vi "HFRR ADV v014 new software.vi"() -> ()   [LabVIEW 2025] (continued)
            n3067 = Concatenate Strings("7)" ("string"), w3910) -> (w3911:string)
            n3068 = Concatenate Strings("8)" ("string"), w3907) -> (w3908:string)
            n3069 = local read "HCF 2"() -> (w3946:dbl)
            n3070 = local read "AVP 2"() -> (w3963:dbl)
            n3071 = local read "s.NO"() -> (w3905:string)
            n3072 = call <vilib>:"New Report.vi"("report type"=enum16{"Standard Report", "HTML"}."Standard Report") -> ("report out"=w3984:refnum<class "NI_report.lvclass">, "error out"=w3983:errorcluster)  [unwired: 13 in]
            n3073 = local read "TITTLE"() -> (w3936:string)
            n3074 = Concatenate Strings(w3961, w3904, w3905, w3961, w3939, w3934, w3961, w3938, w3935, w3961, w3940, w3937, w3961) -> (w3954:string)
            "test by" <- w3954
            n3075 = Number To Fractional String(number=w3960, width (-)=i16 6, precision (6)=i16 2) -> (F-format string=w3949:string)  [unwired: 1 in]
            n3076 = Number To Fractional String(number=w3959, width (-)=i16 6, precision (6)=i16 2) -> (F-format string=w3962:string)  [unwired: 1 in]
            n3077 = Number To Fractional String(number=w3975, width (-)=i16 6, precision (6)=i16 2) -> (F-format string=w3980:string)  [unwired: 1 in]
            n3078 = Number To Fractional String(number=w3964, width (-)=i16 6, precision (6)=i16 2) -> (F-format string=w3966:string)  [unwired: 1 in]
            n3079 = Number To Fractional String(number=w3950, width (-)=i16 6, precision (6)=i16 2) -> (F-format string=w3951:string)  [unwired: 1 in]
            n3080 = Number To Fractional String(number=w3963, width (-)=i16 6, precision (6)=i16 2) -> (F-format string=w3965:string)  [unwired: 1 in]
            n3081 = Number To Fractional String(number=w3946, width (-)=i16 6, precision (6)=i16 2) -> (F-format string=w3945:string)  [unwired: 1 in]
            n3082 = Number To Fractional String(number=w3942, precision (6)=i16 2) -> (F-format string=w3941:string)  [unwired: 2 in]
            n3083 = call-dynamic "Set Report Header Text.vi"("report in"=w3984, "center header text"=w3936, "error in (no error)"=w3983) -> ("report out"=w3955:refnum<class "NI_report.lvclass">, "error out"=w3956:errorcluster)  [unwired: 11 in]
            n3084 = Concatenate Strings(w3944, w3928, w3980, w3944, w3925, w3949, w3944, w3923, w3962, w3944, w3920, w3951, w3944, w3916, w3966, w3944, w3913, w3965, w3944, w3911, w3945, w3944, w3908, w3941) -> (w3932:string)
            "export 2" <- w3932
            n3085 = call-poly <vilib>:"Append Report Text.vi"("report in"=w3955, "text"=w3954, "error in (no error)"=w3956) -> ("report out"=w3958:refnum<class "NI_report.lvclass">, "error out"=w3957:errorcluster)  [unwired: 9 in, 2 out]
            n3086 = local read "test by"() -> (w3931:string)
            n3087 = local read "TITTLE"() -> (w3933:string)
            n3088 = call-poly <vilib>:"Append Report Text.vi"("report in"=w3958, "error in (no error)"=w3957) -> ("report out"=w3979:refnum<class "NI_report.lvclass">, "error out"=w3977:errorcluster)  [unwired: 10 in, 2 out]
            n3089 = Concatenate Strings(w3933, w3932, w3931) -> (→"output":string)
            n3090 = call-poly <vilib>:"Append Report Text.vi"("report in"=w3979, "text"=w3932, "error in (no error)"=w3977) -> ("report out"=w3978:refnum<class "NI_report.lvclass">, "error out"=w3976:errorcluster)  [unwired: 9 in, 2 out]
            n3091 = call-dynamic "Print Report.vi"("report in"=w3978, "printer name (default)"=w3986, "error in (no error)"=w3976) -> ("report out"=w3988:refnum<class "NI_report.lvclass">, "error out"=w3989:errorcluster)  [unwired: 11 in]
            n3092 = call-dynamic "Dispose Report.vi"("report in"=w3988, "error in (no error)"=w3989) -> ()  [unwired: 13 in, 1 out]
          }
        }
        n3093 = case shown="True" "Print 2" {
          frame False {
          }
          frame True {
            n3094 = flat-sequence {
              frame #0 {
                n3095 = local read "s.NO"() -> (→"s.NO 2":string)
                n3096 = Wait (ms)(milliseconds to wait=u32 20) -> ()  [unwired: 1 out]
                n3097 = local read "Sample ID  3"() -> (→"Sample ID  6":string)
                n3098 = local read "Sample ID  4"() -> (→"Sample ID  7":string)
                n3099 = local read "Sample ID"() -> (→"Sample ID  2":string)
                n3100 = local read "Tested by"() -> (→"Tested by 2":string)
                n3101 = local read "Test Date"() -> (→"Test Date 2":string)
                n3102 = local read "Humidity after test 3"() -> (→"Humidity after test 4":dbl)
                n3103 = local read "Ref A Test Date :"() -> (→"TITTLE 4":string)
                n3104 = local read "Temperature before test 3"() -> (w3811:dbl)
                n3105 = local read "Temperature before test 3"() -> (→"Temperature after test 5":dbl)
                n3106 = local read "Temperature after test 3"() -> (→"Temperature after test 4":dbl)
                n3107 = local read "Humidity before test 3"() -> (→"Humidity before test 4":dbl)
                n3108 = local write "Temperature before test 3"(w3811) -> ()
                n3109 = local read "image data"() -> (w3802:T16)
                n3110 = String To Path(string="C:\\LAB-IQ\\im\\Temp_resized.jpg") -> (path=w3803:path)
                "path 2" <- w3803
                n3111 = call <vilib>:"Write JPEG File.vi"("image data"=w3802, "path to JPEG file"=w3803) -> ()  [unwired: 8 in, 2 out]
                "Ref A Test Date :" <- "Ref A Test Date :"
                "Ref B Test Date :" <- "Ref B Test Date :"
                "Ref B Scar Value :" <- "Ref B Scar Value :"
                "Ref A Scar Value :" <- "Ref A Scar Value :"
              }
              frame #1 {
                (unwired) HTML_Report_Image_Alignment."MIDDLE" ("alignment (default)")
                w3839 = u16 0 items=["portrait", "landscape"] ("orientation (portrait)")
                (unwired) HTML_Report_Image_Alignment."ABSMIDDLE" ("alignment (default)")
                (unwired) "TESTED BY : "
                (unwired) "TESTED DATE :"
                (unwired) "SAMPLE ID : "
                (unwired) "SAMPLE DESIGN : "
                w3872 = "\r"
                # "add image"
                n3112 = Wait (ms)(milliseconds to wait=u32 20) -> ()  [unwired: 1 out]
                n3113 = local read "Sample ID  2"() -> (w3865:string)
                n3114 = local read "Wear Scar X"() -> (w3837:dbl)
                "Length ( microns ) 2" <- w3837
                n3115 = local read "Wear Scar Y"() -> (w3836:dbl)
                "Wear Scar Y ( microns ) :" <- w3836
                n3116 = local read "Test Date 2"() -> (w3866:string)
                n3117 = local read "Tested by 2"() -> (w3867:string)
                n3118 = local read "String 46"() -> (w3863:string)
                n3119 = local read "String 48"() -> (w3869:string)
                n3120 = local read "String 47"() -> (w3868:string)
                n3121 = local read "String 49"() -> (w3870:string)
                n3122 = local read "String 10"() -> (w3823:string)
                n3123 = local read "s.NO 2"() -> (w3864:string)
                n3124 = Add(x=w3837, y=w3836) -> (x+y=w3835:dbl)
                n3125 = call <vilib>:"New Report.vi"("report type"=enum16{"Standard Report", "HTML"}."HTML") -> ("report out"=w3843:refnum<class "NI_report.lvclass">, "error out"=w3841:errorcluster)  [unwired: 13 in]
                n3126 = Concatenate Strings(w3872, w3863, w3864, w3872, w3869, w3865, w3872, w3868, w3866, w3872, w3870, w3867, w3872) -> (→"test by 2":string)
                n3127 = Concatenate Strings("C:\\LAB-IQ\\Data\\" ("string"), w3823, ".jpg" ("string")) -> ()  [unwired: 1 out]
                n3128 = Divide(x=w3835, y=2.0) -> (x/y=→"Mean Wear ( microns) :":dbl)
                n3129 = call-dynamic "Set Report Orientation.vi"("report in"=w3843, "orientation (portrait)"=w3839, "error in (no error)"=w3841) -> ("report out"=w3842:refnum<class "NI_report.lvclass">, "error out"=w3840:errorcluster)  [unwired: 11 in]
                n3130 = for {
                  N: 5 -> [_]
                  tunnel: w3842 -> [w3893]
                  tunnel: [w3892] -> w3821
                  tunnel: w3840 -> [w3891]
                  tunnel: [w3890] -> w3820
                  n3131 = call-dynamic "Set Report Tab Width.vi"("report in"=w3893, "error in (no error)"=w3891) -> ("report out"=w3892:refnum<class "NI_report.lvclass">, "error out"=w3890:errorcluster)  [unwired: 12 in]
                }
                n3132 = local read "TITTLE"() -> (w3838:string)
                n3133 = call-dynamic "Set Report Header Text.vi"("report in"=w3821, "center header text"=w3838, "error in (no error)"=w3820) -> ("report out"=w3859:refnum<class "NI_report.lvclass">, "error out"=w3858:errorcluster)  [unwired: 11 in]
                n3134 = for {
                  N: 1 -> [_]
                  tunnel: [w3897] -> w3845
                  tunnel: [w3896] -> w3844
                  tunnel: w3859 -> [w3895]
                  tunnel: w3858 -> [w3894]
                  n3135 = call-dynamic "New Report Line.vi"("report in"=w3895, "error in (no error)"=w3894) -> ("report out"=w3897:refnum<class "NI_report.lvclass">, "error out"=w3896:errorcluster)  [unwired: 12 in]
                }
                n3136 = for {
                  N: 2 -> [_]
                  tunnel: [w3889] -> w3851
                  tunnel: [w3888] -> w3850
                  tunnel: w3845 -> [w3887]
                  tunnel: w3844 -> [w3886]
                  n3137 = call-dynamic "New Report Line.vi"("report in"=w3887, "error in (no error)"=w3886) -> ("report out"=w3889:refnum<class "NI_report.lvclass">, "error out"=w3888:errorcluster)  [unwired: 12 in]
                }
                n3138 = for {
                  N: 25 -> [_]
                  tunnel: w3851 -> [w3885]
                  tunnel: w3850 -> [w3883]
                  tunnel: [w3884] -> w3854
                  tunnel: [w3882] -> w3853
                  n3139 = call-dynamic "Set Report Tab Width.vi"("report in"=w3885, "error in (no error)"=w3883) -> ("report out"=w3884:refnum<class "NI_report.lvclass">, "error out"=w3882:errorcluster)  [unwired: 12 in]
                }
                n3140 = control-ref of="Tab Control 9"() -> (w3849:refnum<vi>)
                n3141 = call-dynamic "Append Control Image to Report.vi"("report in"=w3854, "alignment (default)"=HTML_Report_Image_Alignment."ABSMIDDLE", "ctrl reference"=w3849, "error in (no error)"=w3853) -> ("report out"=w3848:refnum<class "NI_report.lvclass">, "error out"=w3847:errorcluster)  [unwired: 8 in, 2 out]
                n3142 = for {
                  N: 3 -> [_]
                  tunnel: [w3881] -> w3832
                  tunnel: [w3880] -> w3831
                  tunnel: w3848 -> [w3879]
                  tunnel: w3847 -> [w3878]
                  n3143 = call-dynamic "New Report Line.vi"("report in"=w3879, "error in (no error)"=w3878) -> ("report out"=w3881:refnum<class "NI_report.lvclass">, "error out"=w3880:errorcluster)  [unwired: 12 in]
                }
                n3144 = for {
                  N: 100 -> [_]
                  tunnel: w3832 -> [w3877]
                  tunnel: w3831 -> [w3875]
                  tunnel: [w3876] -> w3828
                  tunnel: [w3874] -> w3826
                  n3145 = call-dynamic "Set Report Tab Width.vi"("report in"=w3877, "error in (no error)"=w3875) -> ("report out"=w3876:refnum<class "NI_report.lvclass">, "error out"=w3874:errorcluster)  [unwired: 12 in]
                }
                n3146 = String To Path(string="C:\\LAB-IQ\\im\\Temp_resized.jpg") -> (path=w3818:path)
                n3147 = call-poly <vilib>:"Append Image to Report.vi"("report in"=w3828, "path or URL of image"=w3818, "error in (no error)"=w3826) -> ("report out"=w3827:refnum<class "NI_report.lvclass">, "error out"=w3825:errorcluster)  [unwired: 9 in, 2 out]
                n3148 = call-poly <vilib>:"Open HTML Report in Browser.vi"("report in"=w3827, "error in (no error)"=w3825) -> ("report out"=w3862:refnum<class "NI_report.lvclass">, "error out"=w3861:errorcluster)  [unwired: 11 in, 1 out]
                n3149 = call-dynamic "Dispose Report.vi"("report in"=w3862, "error in (no error)"=w3861) -> ()  [unwired: 13 in, 1 out]
              }
              frame #2 {
              }
              frame #3 {
                n3150 = disable-structure shown="Disabled" {
                  frame Disabled {
                    n3151 = local read "String 10"() -> (w3902:string)
                    n3152 = Concatenate Strings("C:\\LAB-IQ-NXT\\Data\\" ("string"), w3902, ".jpg" ("string")) -> (w3900:string)
                    n3153 = String To Path(string=w3900) -> (path=w3899:path)
                    n3154 = Delete(path (use dialog)=w3899) -> ()  [unwired: 4 in, 3 out]
                  }
                  frame Enabled {
                  }
                }
                n3155 = local write "Print 2"(FALSE ("Print")) -> ()
              }
            }
          }
        }
      }
    }
    n3156 = property on="SetTemp" class="DigNum (strict)"("Disabled"=w1838) -> ()  [unwired: 2 in, 2 out]
    n3157 = Multiply(x=w1828, y=w1830) -> (x*y=w1829:dbl)
    n3158 = local read "MWSD"() -> (w1827:dbl)
    n3159 = Add(x=w1829, y=w1827) -> (x+y=→"WS1.4":dbl)
    n3160 = Wait (ms)(milliseconds to wait=u32 50) -> ()  [unwired: 1 out]
    n3161 = Wait (ms)(milliseconds to wait=u32 50) -> ()  [unwired: 1 out]
    n3162 = local read "Quit"() -> (w1826:bool)
  }
  n3163 = VISA Close(VISA resource name=w52, error in (no error)=w51) -> (error out=w49:errorcluster)
  n3164 = call <vilib>:"Clear Errors.vi"("error in (no error)"=w49) -> ()  [unwired: 5 in, 2 out]
  n3165 = VISA Close(VISA resource name=w37, error in (no error)=w36) -> ()  [unwired: 1 out]
  n3166 = while {
    tunnel: [w4063] -> w46
    shift-right: [w4056] -> _
    shift-left: 0.0 -> [w4059]
    shift-right: [w4055] -> _
    shift-left: 0.0 -> [w4058]
    shift-right: [w4054] -> _
    shift-left: 400.0 ("vc_cmd") -> [w4057]
    stop <- w4063 stop-if-true
    # "PID LOGIC"
    n3167 = local read "RUN"() -> (w4061:bool)
    n3168 = local read "Auto Start Temp"() -> (w4050:bool)
    n3169 = local read "Auto Start Test"() -> (w4060:bool)
    n3170 = local read "START TEMP"() -> (w4052:bool)
    n3171 = And(x=w4050, y=w4060) -> (x .and. y?=w4051:bool)
    n3172 = Or(x=w4061, y=w4051) -> (x .or. y?=w4062:bool)
    n3173 = And(x=w4062, y=w4052) -> (x .and. y?=w4053:bool)
    n3174 = Wait (ms)(milliseconds to wait=u32 20) -> ()  [unwired: 1 out]
    n3175 = case shown="True" w4053 {
      tunnel: [400.0 ("out_vc_cmd") w4083] -> w4054
      tunnel: [w4066 w4085] -> w4055
      tunnel: [w4066 w4084] -> w4056
      tunnel: w4059 -> [_ w4074]
      tunnel: w4058 -> [_ w4073]
      tunnel: w4057 -> [_ w4072]
      frame False {
        w4066 = 0.0 ("error_out")
      }
      frame True {
        n3176 = local read "Set Strk"() -> (w4069:dbl)
        n3177 = local read "LVDT STROKE"() -> (w4067:dbl)
        n3178 = Add(x=w4069, y="Add up Stroke") -> (x+y=w4070:dbl)
        n3179 = formula code="// Zero-Hardcode Explicit Positional-Form PID Engine\n// Inputs: target_stroke, measured_stroke, dt, prev_error, integral_accumulator_in, prev_vc_cmd\n//         kp, ki, kd, max_step_change, max_amplitude, min_amplitude, startup_cmd\n// Outputs: vc_cmd, error_out, out_error, integral_accumulator_out, out_vc_cmd\n\n// 1. Calculate Tracking Error\nfloat current_error = target_stroke - measured_stroke;\nerror_out = current_error;\n\n// 2. Compute Proportional Term\nfloat p_term = kp * current_error;\n\n// 3. Compute Derivative Term\nfloat d_term = 0.0;\nif (dt > 0.0) {\n    d_term = kd * ((current_error - prev_error) / dt);\n}\n\n// 4. Update and Accumulate Integral Term\nfloat current_integral = integral_accumulator_in + (current_error * dt);\nfloat i_term = ki * current_integral;\n\n// 5. Calculate Ideal Target Command\nfloat ideal_command = startup_cmd + p_term + i_term + d_term;\n\n// 6. Anti-Windup Protection (Back-calculation method)\nif (ideal_command > max_amplitude) {\n    float excess = ideal_command - max_amplitude;\n    if (ki > 0.0) {\n        current_integral -= excess / ki;\n    }\n    ideal_command = max_amplitude;\n} else if (ideal_command < min_amplitude) {\n    float excess = ideal_command - min_amplitude;\n    if (ki > 0.0) {\n        current_integral -= excess / ki;\n    }\n    ideal_command = min_amplitude;\n}\n\n// 7. Apply Loop Rate Limiting (Protects voice coil from large voltage steps)\nfloat raw_adjustment = ideal_command - prev_vc_cmd;\n\nif (raw_adjustment > max_step_change) {\n    raw_adjustment = max_step_change;\n} else if (raw_adjustment < -max_step_change) {\n    raw_adjustment = -max_step_change;\n}\n\nfloat next_vc_cmd = prev_vc_cmd + raw_adjustment;\n\n// Final Output Safety Safeguard Clamping\nif (next_vc_cmd > max_amplitude) {\n    next_vc_cmd = max_amplitude;\n} else if (next_vc_cmd < min_amplitude) {\n    next_vc_cmd = min_amplitude;\n}\n\n// 8. Map to Shift Registers for memory persistence\nvc_cmd = next_vc_cmd;\nout_error = current_error;                     \nintegral_accumulator_out = current_integral;  \nout_vc_cmd = next_vc_cmd;"("target_stroke"=w4070, "measured_stroke"=w4067, "dt"="dt", "integral_accumulator_in"=w4073, "prev_error"=w4074, "prev_vc_cmd"=w4072, "kp"="kp", "ki"="ki", "kd"="kd", "max_step_change"="max_step_change", "max_amplitude"="max_amplitude", "min_amplitude"="min_amplitude", "startup_cmd"="startup_cmd") -> ("vc_cmd"=w4089:dbl, "out_error"=w4084:dbl, "integral_accumulator_out"=w4085:dbl, "out_vc_cmd"=w4083:dbl)  [unwired: 1 out]
        "output Vpp" <- w4089
        n3180 = Number To Fractional String(number=w4089, precision (6)=i16 1) -> (F-format string=w4087:string)  [unwired: 2 in]
        n3181 = Concatenate Strings("DAC;" ("string"), w4087) -> (w4071:string)
        n3182 = local write "Command"(w4071) -> ()
        "prev_error" <- w4074
        "integral_accumulator_in" <- w4073
        "prev_vc_cmd" <- w4072
      }
    }
    n3183 = local read "Quit"() -> (w4063:bool)
  }
  n3184 = Or(x=w42, y=w41) -> (x .or. y?=w43:bool)
  n3185 = Or(x=w39, y=w43) -> (x .or. y?=w48:bool)
  n3186 = control-ref of="new picture"() -> ()  [unwired: 1 out]
  n3187 = Or(x=w54, y=w48) -> (x .or. y?=w45:bool)
  n3188 = Or(x=w45, y=w46) -> (x .or. y?=w40:bool)
  n3189 = while {
    tunnel: [w4090] -> w53
    i -> [w4097]
    stop <- w4090 stop-if-true
    n3190 = local read "Quit"() -> (w4090:bool)
    n3191 = Equal To 0?(x=w4097) -> (x = 0?=w4095:bool)
    n3192 = call "Elapsed Time3"("Time Target (s)"=45.0, "Auto Reset"=TRUE) -> ("Time has Elapsed"=w4094:bool)  [unwired: 10 in, 7 out]
    n3193 = Wait (ms)(milliseconds to wait=u32 50) -> ()  [unwired: 1 out]
    n3194 = Or(x=w4094, y=w4095) -> (x .or. y?=w4096:bool)
    n3195 = case shown="True" w4096 {
      frame False {
      }
      frame True {
        n3196 = call <vilib>:"System Exec.vi"("run minimized? (F)"=TRUE, "error in (no error)"="error in (no error)", "command line"="powercfg.exe -change -monitor-timeout-ac 0") -> ("error out"=w4108:errorcluster)  [unwired: 5 in, 3 out]
        n3197 = call <vilib>:"System Exec.vi"("run minimized? (F)"=TRUE, "error in (no error)"=w4108, "command line"="powercfg.exe -change -disk-timeout-ac 0") -> ("error out"=w4107:errorcluster)  [unwired: 5 in, 3 out]
        n3198 = call <vilib>:"System Exec.vi"("run minimized? (F)"=TRUE, "error in (no error)"=w4107, "command line"="powercfg.exe -change -standby-timeout-ac 0") -> ("error out"=w4106:errorcluster)  [unwired: 5 in, 3 out]
        n3199 = call <vilib>:"System Exec.vi"("run minimized? (F)"=TRUE, "error in (no error)"=w4106, "command line"="powercfg.exe -change -hibernate-timeout-ac 0") -> ("error out"=w4105:errorcluster)  [unwired: 5 in, 3 out]
        n3200 = call <vilib>:"Simple Error Handler.vi"("error in (no error)"=w4105) -> ("error out"=w4111:errorcluster)  [unwired: 4 in, 4 out]
        n3201 = call <vilib>:"Clear Errors.vi"("error in (no error)"=w4111) -> ("error out"=→"error out":errorcluster)  [unwired: 5 in, 1 out]
      }
    }
  }
  n3202 = Compound Arithmetic op=OR(w56, w40, w53) -> (w55:bool)
  n3203 = flat-sequence {
    tunnel: w55 -> [_]
    tunnel: [w4113] -> w18
    tunnel: w18 -> [_]
    frame #0 {
      n3204 = call "CLOSE CONNECTION.vi"() -> ("error out"=w4113:errorcluster)  [unwired: 11 in]
    }
    frame #1 {
      n3205 = Quit LabVIEW(quit? (T)=TRUE) -> ()
      n3206 = local write "Quit"(FALSE ("EXIT")) -> ()
    }
  }
  n3207 = property on="Heater Button" class="Bool (strict)"("Visible"=TRUE) -> ()  [unwired: 2 in, 2 out]
  n3208 = disable-structure shown="Disabled" {
    disable-tunnel: _ -> [w4119 _]
    disable-tunnel: _ -> [w4116 _]
    disable-tunnel: _ -> [w4117 _]
    frame Disabled {
      n3209 = disable-structure shown="Disabled" {
        disable-tunnel: [w4126 _] -> w4118
        frame Disabled {
          n3210 = while {
            shift-right: [w4168] -> w4124
            shift-left: errorcluster {"status"=TRUE, "code"=0, "source"="Init"} ("error out") -> [w4133]
            shift-right: [w4167] -> w4123
            shift-left: _ -> [w4134]
            shift-right: [w4166] -> _
            shift-left: "" -> [w4165]
            tunnel: [w4127] -> w4126
            shift-right: ["Set Rh"] -> _
            shift-left: 0.0 ("Set Rh") -> [w4159]
            tunnel: [w4136] -> _
            i -> [w4136]
            stop <- w4127 stop-if-true
            n3211 = flat-sequence {
              tunnel: w4133 -> [w4171]
              tunnel: [w4171] -> w4132
              frame #0 {
                n3212 = Wait (ms)(milliseconds to wait=u32 200) -> ()  [unwired: 1 out]
              }
            }
            n3213 = local read "Com Port 3"() -> (w4135:refnum<visa-resource-name>)
            n3214 = local read "Humidity Str Rec"() -> (w4137:string)
            n3215 = Not Equal?(x="Set Rh", y=w4159) -> (x != y?=w4164:bool)
            n3216 = Number To Decimal String(number="Set Rh") -> (decimal integer string=w4162:string)  [unwired: 1 in]
            n3217 = Not Equal?(x=w4135, y=w4134) -> (x != y?=w4130:bool)
            n3218 = Concatenate Strings("#setPoint00" ("string"), w4162) -> (w4163:string)
            n3219 = case shown="False" w4164 {
              tunnel: w4163 -> [_ w4183]
              frame False {
                n3220 = local read "Humidity"() -> (w4180:bool)
                n3221 = case shown="True" w4180 {
                  frame False {
                    n3222 = local write "Humidity Str Send"("stop" ("Humidity Str Send")) -> ()
                  }
                  frame True {
                    n3223 = local write "Humidity Str Send"("start" ("Humidity Str Send")) -> ()
                  }
                }
              }
              frame True {
                n3224 = local write "Humidity Str Send"(w4183) -> ()
              }
            }
            n3225 = Or(x=w4130) -> (y=w4128:bool, x .or. y?=w4129:bool)
            n3226 = String Subset(string=w4137, offset (0)=7) -> (substring=w4152:string)  [unwired: 1 in]
            n3227 = Match Pattern(string=w4137, regular expression="?") -> (offset past match=w4155:i32)  [unwired: 1 in, 3 out]
            n3228 = Match Pattern(string=w4137, regular expression="v") -> (offset past match=w4158:i32)  [unwired: 1 in, 3 out]
            n3229 = case shown="True" w4129 {
              tunnel: w4132 -> [w4169 _]
              tunnel: [w4169 errorcluster {"status"=TRUE, "code"=0, "source"="Init"} ("error out")] -> w4131
              frame False {
              }
              frame True {
              }
            }
            n3230 = Equal?(x=w4155, y=-1) -> (x = y?=w4139:bool)
            n3231 = Match Pattern(string=w4152, regular expression="g") -> (after substring=w4153:string, offset past match=w4144:i32)  [unwired: 1 in, 2 out]
            n3232 = Match Pattern(string=w4152, regular expression="y") -> (after substring=w4151:string, offset past match=w4145:i32)  [unwired: 1 in, 2 out]
            n3233 = Greater?(x=w4145, y=w4144) -> (0:w4150:bool)
            n3234 = Greater Or Equal To 0?(x=w4145) -> (x >= 0?=w4142:bool)
            n3235 = Greater Or Equal To 0?(x=w4144) -> (x >= 0?=w4143:bool)
            n3236 = Or(x=w4142, y=w4143) -> (x .or. y?=w4141:bool)
            n3237 = Greater Or Equal To 0?(x=w4158) -> (x >= 0?=w4140:bool)
            n3238 = Select(t=w4151, s=w4150, f=w4153) -> (s? t:f=w4146:string)
            n3239 = case shown="Error" w4131 {
              selector: w4131 -> [w4196 w4242]
              tunnel: [w4194 w4235] -> w4168
              tunnel: w4134 -> [w4197 w4241]
              tunnel: [w4195 w4244] -> w4167
              tunnel: w4165 -> [w4184 w4243]
              tunnel: [w4191 w4243] -> w4166
              frame No Error {
                n3240 = call "Elapsed Time7"() -> ("Time has Elapsed"=w4190:bool)  [unwired: 12 in, 7 out]
                n3241 = Not Equal?(x="Humidity Str Send", y=w4184) -> (x != y?=w4186:bool)
                n3242 = Or(x=w4186, y=w4190) -> (x .or. y?=w4189:bool)
                n3243 = Select(t="Humidity Str Send", s=w4186, f="vals" ("regular expression")) -> (s? t:f=w4185:string)
                n3244 = Or(x=w4189, y="Send") -> (x .or. y?=w4193:bool)
                n3245 = case shown="True" w4193 {
                  tunnel: [w4200 w4205] -> w4194
                  tunnel: w4197 -> [w4199 w4213]
                  tunnel: w4196 -> [w4200 w4212]
                  tunnel: [w4199 w4206] -> w4195
                  tunnel: w4185 -> [_ w4211]
                  tunnel: [w4198 w4202] -> w4191
                  tunnel: "Humidity Str Send" -> [_ w4203]
                  tunnel: w4186 -> [_ w4204]
                  tunnel: w4184 -> [w4198 w4201]
                  frame False {
                  }
                  frame True {
                    n3246 = flat-sequence {
                      tunnel: w4213 -> [w4221]
                      tunnel: w4212 -> [w4220]
                      tunnel: w4211 -> [w4217]
                      tunnel: [w4219] -> w4210
                      tunnel: [w4218] -> w4209
                      tunnel: w4210 -> [w4224]
                      tunnel: w4209 -> [w4223]
                      tunnel: [w4224] -> w4208
                      tunnel: [w4223] -> w4207
                      tunnel: w4208 -> [w4231]
                      tunnel: w4207 -> [w4230]
                      tunnel: [w4229] -> w4206
                      tunnel: [w4228] -> w4205
                      frame #0 {
                        n3247 = local write "Ser Led"(TRUE ("Boolean 4")) -> ()
                        n3248 = Concatenate Strings(w4217, "\r") -> (w4216:string)
                        n3249 = VISA Write(VISA resource name=w4221, write buffer=w4216, error in (no error)=w4220) -> (VISA resource name out=w4219:refnum<visa-resource-name>, error out=w4218:errorcluster)  [unwired: 1 out]
                      }
                      frame #1 {
                        n3250 = Wait (ms)(milliseconds to wait="wait") -> ()  [unwired: 1 out]
                      }
                      frame #2 {
                        w4226 = FALSE ("Send")
                        n3251 = property class="Instr"(reference=w4231, error in=w4230) -> (reference out=w4232:refnum<visa-resource-name>, error out=w4233:errorcluster, "Serial Settings:Number of Bytes at Serial Port"=w4225:u32)
                        n3252 = local write "Send"(w4226) -> ()
                        n3253 = local write "Ser Led"(w4226) -> ()
                        n3254 = VISA Read(VISA resource name=w4232, byte count=w4225, error in (no error)=w4233) -> (VISA resource name out=w4229:refnum<visa-resource-name>, read buffer=→"Humidity Str Rec":string, error out=w4228:errorcluster)  [unwired: 1 out]
                      }
                    }
                    n3255 = Select(t=w4203, s=w4204, f=w4201) -> (s? t:f=w4202:string)
                  }
                }
              }
              frame Error {
                w4249 = u16 0 items=["None"=0, "XON/XOFF"=1, "RTS/CTS"=2, "DTR/DSR"=4] ("flow control")
                w4245 = u16 0 items=["None", "Odd", "Even", "Mark", "Space"] ("parity")
                w4248 = u16 10 items=["1.0"=10, "1.5"=15, "2.0"=20] ("stop bits")
                n3256 = VISA Close(VISA resource name=w4241, error in (no error)=w4242) -> (error out=w4240:errorcluster)
                n3257 = local write "humid"("" ("humid")) -> ()
                n3258 = local write "Humidity Str Rec"("" ("Humidity Str Rec")) -> ()
                n3259 = call <vilib>:"Clear Errors.vi"("error in (no error)"=w4240) -> ("error out"=w4239:errorcluster)  [unwired: 5 in, 1 out]
                n3260 = local read "Com Port 3"() -> (w4238:refnum<visa-resource-name>)
                n3261 = call-poly "VISA Configure Serial Port"("VISA resource name"=w4238, "timeout (10sec)"=u32 1000, "termination char\n(0xA = '\\n' = LF)"=u8 10 ("termination char\n(0xA = '\\n' = LF)"), "Enable Termination\nChar (T)"=FALSE ("Enable Termination Char (T)"), "data bits (8)"=u16 8 ("data bits"), "parity (0:none)"=w4245, "error in (no error)"=w4239, "stop bits (10: 1 bit)"=w4248, "flow control (0:none)"=w4249) -> ("VISA resource name out"=w4244:refnum<visa-resource-name>, "baud rate (9600)"=w4236:u32, "error out"=w4235:errorcluster)  [unwired: 4 in]
              }
            }
            n3262 = Compound Arithmetic op=AND(w4140, w4139, w4141) -> (w4138:bool)
            n3263 = case shown="True" w4138 {
              tunnel: w4137 -> [_ _]
              tunnel: w4146 -> [_ w4176]
              frame False {
              }
              frame True {
                w4174 = " " ("regular expression")
                n3264 = Match Pattern(string=w4176, regular expression=" ") -> (after substring=w4178:string)  [unwired: 1 in, 3 out]
                n3265 = Match Pattern(string=w4178, regular expression=w4174) -> (before substring=→"humid":string, after substring=w4175:string)  [unwired: 1 in, 2 out]
                n3266 = Match Pattern(string=w4175, regular expression=w4174) -> (before substring=→"temp_@Rh sensor":string)  [unwired: 1 in, 3 out]
              }
            }
            n3267 = local read "Quit"() -> (w4127:bool)
          }
          n3268 = VISA Close(VISA resource name=w4123, error in (no error)=w4124) -> (error out=w4120:errorcluster)
          n3269 = call <vilib>:"Clear Errors.vi"("error in (no error)"=w4120) -> ()  [unwired: 5 in, 2 out]
        }
        frame Enabled {
        }
      }
    }
    frame Enabled {
    }
  }
  n3270 = while {
    tunnel: [w4256] -> _
    i -> [w4256]
    stop <- w4252 stop-if-true
    # "Langauage selection"
    n3271 = Equal?(x="Lan flag", y=22.0) -> ()  [unwired: 1 out]
    n3272 = disable-structure shown="Disabled" {
      frame Disabled {
        n3273 = stacked-sequence {
          frame #0 {
            n3274 = case shown="\"Russian\"" "Language Selection" {
              tunnel: [0 1] -> w4258
              frame "English", Default {
              }
              frame "Russian" {
              }
            }
            n3275 = for {
              N: 130 -> [_]
              tunnel: "Table" -> [w4267]
              tunnel: w4258 -> [w4266]
              i -> [w4265]
              n3276 = Index Array(array=w4267, index (row)=w4265, index (col)=w4266) -> (element=w4264:string)
              n3277 = case shown="123" w4265 {
                tunnel: w4264 -> [w4268 w4269 _ w4270 w4271 w4272 w4273 w4274 w4275 w4276 w4277 w4278 w4279 w4280 w4281 w4282 w4283 w4284 w4285 w4286 w4287 w4288 w4289 w4290 w4291 w4292 w4293 w4294 w4295 _ _ w4296 w4297 w4298 w4299 w4300 w4301 w4310 w4317 w4324 w4331 w4335 w4338 w4341 w4343 w4345 w4346 w4347 w4348 w4349 w4350 w4351 w4352 w4353 w4354 w4355 w4356 w4357 w4358 w4359 w4360 w4361 w4362 w4363 w4364 w4365 w4366 w4367 w4368 w4369 w4370 w4371 w4372 w4373 w4374 w4375 w4376 w4377 w4378 w4379 w4380 w4381 w4382 w4383 w4384 w4385 w4386 w4387 w4388 w4389 w4390 w4391 w4392 w4393 w4394 w4395 w4396 w4397 w4398 w4399 w4400 w4401 w4402 w4403 w4404 _ w4405 w4406 w4407 w4408 w4409 w4410 w4411 w4412 w4413 w4414 w4415 w4416 w4417 _ w4418 w4419 w4420 w4421 w4422 w4423 _]
                frame 0 {
                  n3278 = local write "S"(w4268) -> ()
                }
                frame 1 {
                  n3279 = local write "S 2"(w4269) -> ()
                }
                frame 2 {
                }
                frame 3 {
                  n3280 = local write "S 4"(w4270) -> ()
                }
                frame 4 {
                  n3281 = property on="FILE" class="Str"("Caption.Text"=w4271) -> ()  [unwired: 2 in, 2 out]
                }
                frame 5 {
                  n3282 = property on="Fuel Discription :" class="Str"("Caption.Text"=w4272) -> ()  [unwired: 2 in, 2 out]
                }
                frame 6 {
                  n3283 = property on="Remarks :" class="Str"("Caption.Text"=w4273) -> ()  [unwired: 2 in, 2 out]
                }
                frame 7 {
                  n3284 = property on="Save & Continue" class="Bool (strict)"("Boolean Text.Text"=w4274) -> ()  [unwired: 2 in, 2 out]
                }
                frame 8 {
                }
                frame 9 {
                  n3285 = property on="Set Hz" class="DigNum (strict)"("Caption.Text"=w4276) -> ()  [unwired: 2 in, 2 out]
                }
                frame 10 {
                  "String 3" <- w4277
                }
                frame 11 {
                  n3286 = property on="NORMAL LOAD" class="DigNum (strict)"("Caption.Text"=w4278) -> ()  [unwired: 2 in, 2 out]
                }
                frame 12 {
                  "String 5" <- w4279
                }
                frame 13 {
                  n3287 = property on="Set Temp" class="DigNum (strict)"("Caption.Text"=w4280) -> ()  [unwired: 2 in, 2 out]
                }
                frame 14 {
                  n3288 = local write "S 15"(w4281) -> ()
                }
                frame 15 {
                  n3289 = property on="Set Rh" class="DigNum (strict)"("Caption.Text"=w4282) -> ()  [unwired: 2 in, 2 out]
                }
                frame 16 {
                  "String 13" <- w4283
                  "String 26" <- w4283
                }
                frame 17 {
                  n3290 = local write "S 18"(w4284) -> ()
                }
                frame 18 {
                  "String 17" <- w4285
                }
                frame 19 {
                  n3291 = property on="test time" class="DigNum (strict)"("Caption.Text"=w4286) -> ()  [unwired: 2 in, 2 out]
                }
                frame 20 {
                  "String 18" <- w4287
                  "String 22" <- w4287
                }
                frame 21 {
                  n3292 = property on="Elapsed time" class="DigNum (strict)"("Caption.Text"=w4288) -> ()  [unwired: 2 in, 2 out]
                }
                frame 22 {
                  n3293 = property on="Samplingtime 2" class="DigNum (strict)"("Caption.Text"=w4289) -> ()  [unwired: 2 in, 2 out]
                }
                frame 23 {
                  "String 21" <- w4290
                }
                frame 24 {
                  n3294 = property on="Countdown" class="DigNum (strict)"("Caption.Text"=w4291) -> ()  [unwired: 2 in, 2 out]
                }
                frame 25 {
                  n3295 = property on="Countdown 2" class="DigNum (strict)"("Caption.Text"=w4292) -> ()  [unwired: 2 in, 2 out]
                }
                frame 26 {
                  n3296 = property on="Engage" class="Bool (strict)"("Boolean Text.Text"=w4293) -> ()  [unwired: 2 in, 2 out]
                }
                frame 27 {
                  n3297 = property on="Boolean  4" class="Bool (strict)"("Boolean Text.Text"=w4294) -> ()  [unwired: 2 in, 2 out]
                }
                frame 28 {
                  n3298 = property on="Test \nStatus" class="Bool (strict)"("Boolean Text.Text"=w4295) -> ()  [unwired: 2 in, 2 out]
                }
                frame 29 {
                }
                frame 30 {
                }
                frame 31 {
                }
                frame 32 {
                  n3299 = property on="RSTCOF" class="Bool"("Boolean Text.Text"=w4297) -> ()  [unwired: 2 in, 2 out]
                  n3300 = property on="RST FF" class="Bool"("Boolean Text.Text"=w4297) -> ()  [unwired: 2 in, 2 out]
                  n3301 = property on="RST TEMP" class="Bool"("Boolean Text.Text"=w4297) -> ()  [unwired: 2 in, 2 out]
                  n3302 = property on="RSTV1 3" class="Bool"("Boolean Text.Text"=w4297) -> ()  [unwired: 2 in, 2 out]
                  n3303 = property on="rstv2" class="Bool"("Boolean Text.Text"=w4297) -> ()  [unwired: 2 in, 2 out]
                  n3304 = property on="RSTV1 2" class="Bool"("Boolean Text.Text"=w4297) -> ()  [unwired: 2 in, 2 out]
                  n3305 = property on="RST CP" class="Bool"("Boolean Text.Text"=w4297) -> ()  [unwired: 2 in, 2 out]
                }
                frame 33 {
                  "S 61" <- w4298
                }
                frame 34 {
                  "String 23" <- w4299
                }
                frame 35 {
                  n3306 = property on="Rh Before" class="DigNum (strict)"("Caption.Text"=w4300) -> ()  [unwired: 2 in, 2 out]
                }
                frame 36 {
                  n3307 = Match Pattern(string=w4301, regular expression=",") -> (before substring=→"bs":string, after substring=→"as":string)  [unwired: 1 in, 2 out]
                  n3308 = property on="Rh After" class="DigNum (strict)"("Caption.Text"=w4301) -> ()  [unwired: 2 in, 2 out]
                }
                frame 37 {
                  n3309 = Match Pattern(string=w4310, regular expression=",") -> (before substring=w4309:string, after substring=w4308:string)  [unwired: 1 in, 2 out]
                  "bs" <- w4309
                  "as" <- w4308
                  n3310 = Concatenate Strings(w4309, w4308) -> (w4305:string)
                  n3311 = property on="Humidity before test 2" class="DigNum (strict)"("Caption.Text"=w4305) -> ()  [unwired: 2 in, 2 out]
                  n3312 = property on="Humidity before test" class="DigNum (strict)"("Caption.Text"=w4305) -> ()  [unwired: 2 in, 2 out]
                  n3313 = Concatenate Strings(w4305, "=" ("string")) -> (w4306:string)
                  n3314 = local write "S 38"(w4306) -> ()
                }
                frame 38 {
                  n3315 = Match Pattern(string=w4317, regular expression=",") -> (before substring=w4316:string, after substring=w4315:string)  [unwired: 1 in, 2 out]
                  "bs" <- w4316
                  "as" <- w4315
                  n3316 = Concatenate Strings(w4316, w4315) -> (w4312:string)
                  n3317 = property on="Humidity after test 2" class="DigNum (strict)"("Caption.Text"=w4312) -> ()  [unwired: 2 in, 2 out]
                  n3318 = Concatenate Strings(w4312, "=" ("string")) -> (w4314:string)
                  n3319 = property on="Humidity after test" class="DigNum (strict)"("Caption.Text"=w4312) -> ()  [unwired: 2 in, 2 out]
                  n3320 = local write "S 39"(w4314) -> ()
                }
                frame 39 {
                  n3321 = Match Pattern(string=w4324, regular expression=",") -> (before substring=w4323:string, after substring=w4322:string)  [unwired: 1 in, 2 out]
                  "bs" <- w4323
                  "as" <- w4322
                  n3322 = Concatenate Strings(w4323, w4322) -> (w4319:string)
                  n3323 = property on="Temperature before test 2" class="DigNum (strict)"("Caption.Text"=w4319) -> ()  [unwired: 2 in, 2 out]
                  n3324 = property on="Temperature before test" class="DigNum (strict)"("Caption.Text"=w4319) -> ()  [unwired: 2 in, 2 out]
                  n3325 = Concatenate Strings(w4319, "=" ("string")) -> (→"String 34":string)
                }
                frame 40 {
                  n3326 = Match Pattern(string=w4331, regular expression=",") -> (before substring=w4330:string, after substring=w4329:string)  [unwired: 1 in, 2 out]
                  "bs" <- w4330
                  "as" <- w4329
                  n3327 = Concatenate Strings(w4330, w4329) -> (w4326:string)
                  n3328 = property on="Temperature after test 2" class="DigNum (strict)"("Caption.Text"=w4326) -> ()  [unwired: 2 in, 2 out]
                  n3329 = Concatenate Strings(w4326, "=" ("string")) -> (→"String 35":string)
                  n3330 = property on="Temperature after test" class="DigNum (strict)"("Caption.Text"=w4326) -> ()  [unwired: 2 in, 2 out]
                }
                frame 41 {
                  n3331 = property on="AVP" class="DigNum (strict)"("Caption.Text"=w4335) -> ()  [unwired: 2 in, 2 out]
                  n3332 = property on="AVP 2" class="DigNum (strict)"("Caption.Text"=w4335) -> ()  [unwired: 2 in, 2 out]
                  n3333 = Concatenate Strings(w4335, "=" ("string")) -> (→"String 36":string)
                }
                frame 42 {
                  n3334 = property on="MWSD" class="DigNum (strict)"("Caption.Text"=w4338) -> ()  [unwired: 2 in, 2 out]
                  n3335 = property on="MWSD 2" class="DigNum (strict)"("Caption.Text"=w4338) -> ()  [unwired: 2 in, 2 out]
                  n3336 = Concatenate Strings(w4338, "=" ("string")) -> (→"String 37":string)
                }
                frame 43 {
                  n3337 = property on="HCF 2" class="DigNum (strict)"("Caption.Text"=w4341) -> ()  [unwired: 2 in, 2 out]
                  n3338 = property on="HCF" class="DigNum (strict)"("Caption.Text"=w4341) -> ()  [unwired: 2 in, 2 out]
                  n3339 = Concatenate Strings(w4341, "=" ("string")) -> (→"String 38":string)
                }
                frame 44 {
                  n3340 = Concatenate Strings(w4343, "=" ("string")) -> (→"String 39":string)
                  n3341 = property on="WS1.4 2" class="DigNum (strict)"("Caption.Text"=w4343) -> ()  [unwired: 2 in, 2 out]
                  n3342 = property on="WS1.4" class="DigNum (strict)"("Caption.Text"=w4343) -> ()  [unwired: 2 in, 2 out]
                }
                frame 45 {
                  n3343 = property on="Save Results" class="Bool (strict)"("Boolean Text.Text"=w4345) -> ()  [unwired: 2 in, 2 out]
                }
                frame 46 {
                  n3344 = local write "S 47"(w4346) -> ()
                }
                frame 47 {
                  n3345 = local write "S 48"(w4347) -> ()
                }
                frame 48 {
                  n3346 = local write "S 49"(w4348) -> ()
                }
                frame 49 {
                  n3347 = local write "S 50"(w4349) -> ()
                }
                frame 50 {
                  n3348 = local write "S 51"(w4350) -> ()
                }
                frame 51 {
                  n3349 = local write "S 52"(w4351) -> ()
                }
                frame 52 {
                  n3350 = local write "S 53"(w4352) -> ()
                }
                frame 53 {
                  n3351 = local write "S 54"(w4353) -> ()
                }
                frame 54 {
                  n3352 = local write "S 55"(w4354) -> ()
                }
                frame 55 {
                  n3353 = local write "S 56"(w4355) -> ()
                }
                frame 56 {
                  n3354 = local write "S 57"(w4356) -> ()
                }
                frame 57 {
                  n3355 = local write "S 58"(w4357) -> ()
                }
                frame 58 {
                  n3356 = local write "S 59"(w4358) -> ()
                }
                frame 59 {
                  n3357 = local write "S 60"(w4359) -> ()
                }
                frame 60 {
                  n3358 = local write "S 62"(w4360) -> ()
                }
                frame 61 {
                  n3359 = local write "S 63"(w4361) -> ()
                }
                frame 62 {
                  n3360 = local write "S 64"(w4362) -> ()
                }
                frame 63 {
                  n3361 = local write "S 65"(w4363) -> ()
                }
                frame 64 {
                  n3362 = local write "S 66"(w4364) -> ()
                }
                frame 65 {
                  n3363 = local write "S 67"(w4365) -> ()
                }
                frame 66 {
                  n3364 = local write "S 68"(w4366) -> ()
                }
                frame 67 {
                  n3365 = local write "S 69"(w4367) -> ()
                }
                frame 68 {
                  n3366 = local write "S 70"(w4368) -> ()
                }
                frame 69 {
                  n3367 = local write "S 71"(w4369) -> ()
                }
                frame 70 {
                  n3368 = local write "S 72"(w4370) -> ()
                }
                frame 71 {
                  n3369 = local write "S 73"(w4371) -> ()
                }
                frame 72 {
                  n3370 = local write "S 74"(w4372) -> ()
                }
                frame 73 {
                  n3371 = local write "S 75"(w4373) -> ()
                }
                frame 74 {
                  n3372 = local write "S 76"(w4374) -> ()
                }
                frame 75 {
                  n3373 = local write "S 77"(w4375) -> ()
                }
                frame 76 {
                  n3374 = local write "S 78"(w4376) -> ()
                }
                frame 77 {
                  n3375 = local write "S 79"(w4377) -> ()
                }
                frame 79 {
                  n3376 = property on="Sample Temperature ( °C )" class="XYGraph (strict)"("Y Scale.Name Label.Text"=w4378) -> ()  [unwired: 2 in, 2 out]
                }
                frame 80 {
                  n3377 = local write "S 81"(w4379) -> ()
                  n3378 = property on="Humidity ( %RH )" class="XYGraph (strict)"("Y Scale.Name Label.Text"=w4379) -> ()  [unwired: 2 in, 2 out]
                }
                frame 78 {
                  n3379 = property on="Air Temperature  ( °C )" class="XYGraph (strict)"("X Scale.Name Label.Text"=w4380) -> ()  [unwired: 2 in, 2 out]
                  n3380 = property on="Humidity ( %RH )" class="XYGraph (strict)"("X Scale.Name Label.Text"=w4380) -> ()  [unwired: 2 in, 2 out]
                  n3381 = property on="Sample Temperature ( °C )" class="XYGraph (strict)"("X Scale.Name Label.Text"=w4380) -> ()  [unwired: 2 in, 2 out]
                  n3382 = property on="Coefficient Of Friction" class="XYGraph (strict)"("X Scale.Name Label.Text"=w4380) -> ()  [unwired: 2 in, 2 out]
                }
                frame 81 {
                  n3383 = property on="Air Temperature  ( °C )" class="XYGraph (strict)"("Y Scale.Name Label.Text"=w4381) -> ()  [unwired: 2 in, 2 out]
                }
                frame 82 {
                  n3384 = local write "S 84"(w4382) -> ()
                }
                frame 83 {
                  n3385 = local write "S 85"(w4383) -> ()
                }
                frame 84 {
                  n3386 = local write "S 86"(w4384) -> ()
                }
                frame 85 {
                  n3387 = local write "S 87"(w4385) -> ()
                }
                frame 86 {
                  n3388 = local write "S 88"(w4386) -> ()
                }
                frame 87 {
                }
                frame 88 {
                  n3389 = local write "S 90"(w4388) -> ()
                }
                frame 89 {
                  n3390 = local write "S 91"(w4389) -> ()
                }
                frame 90 {
                  n3391 = local write "S 92"(w4390) -> ()
                }
                frame 91 {
                  n3392 = local write "S 93"(w4391) -> ()
                }
                frame 92 {
                  n3393 = local write "S 94"(w4392) -> ()
                }
                frame 93 {
                  n3394 = local write "S 95"(w4393) -> ()
                }
                frame 94 {
                  n3395 = local write "S 96"(w4394) -> ()
                }
                frame 95 {
                  n3396 = local write "S 97"(w4395) -> ()
                }
                frame 96 {
                  n3397 = local write "S 98"(w4396) -> ()
                }
                frame 97 {
                  n3398 = local write "S 99"(w4397) -> ()
                }
                frame 98 {
                  n3399 = local write "S 100"(w4398) -> ()
                }
                frame 99 {
                  n3400 = local write "S 101"(w4399) -> ()
                }
                frame 100 {
                  n3401 = local write "S 102"(w4400) -> ()
                }
                frame 101 {
                  n3402 = local write "S 103"(w4401) -> ()
                }
                frame 102 {
                  n3403 = local write "S 104"(w4402) -> ()
                }
                frame 103 {
                  n3404 = local write "S 105"(w4403) -> ()
                }
                frame 104 {
                  n3405 = local write "S 106"(w4404) -> ()
                }
                frame 105 {
                }
                frame 106 {
                  n3406 = property on="OK Button 17" class="Bool (strict)"("Boolean Text.Text"=w4405) -> ()  [unwired: 2 in, 2 out]
                }
                frame 107 {
                  n3407 = property on="OK Button 16" class="Bool (strict)"("Boolean Text.Text"=w4406) -> ()  [unwired: 2 in, 2 out]
                }
                frame 108 {
                  n3408 = property on="TITTLE" class="Str"("Caption.Text"=w4407) -> ()  [unwired: 2 in, 2 out]
                }
                frame 109 {
                  "String 30" <- w4408
                }
                frame 110 {
                  n3409 = property on="Test Date" class="Str"("Caption.Text"=w4409) -> ()  [unwired: 2 in, 2 out]
                  "String 31" <- w4409
                }
                frame 111 {
                  n3410 = property on="Sample ID" class="Str"("Caption.Text"=w4410) -> ()  [unwired: 2 in, 2 out]
                  "String 32" <- w4410
                }
                frame 112 {
                  n3411 = property on="Tested by" class="Str"("Caption.Text"=w4411) -> ()  [unwired: 2 in, 2 out]
                  "String 33" <- w4411
                }
                frame 113 {
                  n3412 = property on="System Configured Printers 2" class="Arr (strict)"("Caption.Text"=w4412) -> ()  [unwired: 2 in, 2 out]
                }
                frame 114 {
                  n3413 = property on="Selected Printer" class="Str"("Caption.Text"=w4413) -> ()  [unwired: 2 in, 2 out]
                }
                frame 115 {
                  n3414 = property on="Select Printer 3" class="DigNum (strict)"("Caption.Text"=w4414) -> ()  [unwired: 2 in, 2 out]
                }
                frame 116 {
                  n3415 = property on="Print" class="Bool (strict)"("Boolean Text.Text"=w4415) -> ()  [unwired: 2 in, 2 out]
                }
                frame 117 {
                  "String 41" <- w4416
                }
                frame 118 {
                  n3416 = property on="tested by" class="Str"("Caption.Text"=w4417) -> ()  [unwired: 2 in, 2 out]
                }
                frame 119 {
                }
                frame 120 {
                  n3417 = property on="Export" class="Bool (strict)"("Boolean Text.Text"=w4418) -> ()  [unwired: 2 in, 2 out]
                }
                frame 121 {
                  n3418 = property on="TEMP INTERCEPT:" class="DigNum (strict)"("Caption.Text"=w4419) -> ()  [unwired: 2 in, 2 out]
                }
                frame 122 {
                  n3419 = property on="AIR TEMP INTERCEPT:" class="DigNum (strict)"("Caption.Text"=w4420) -> ()  [unwired: 2 in, 2 out]
                }
                frame 123 {
                  n3420 = property on="Select File Type" class="Enum (strict)"("Caption.Text"=w4421) -> ()  [unwired: 2 in, 2 out]
                }
                frame 124 {
                  n3421 = property on="s.NO" class="Str"("Caption.Text"=w4422) -> ()  [unwired: 2 in, 2 out]
                  "String 45" <- w4422
                }
                frame 125 {
                  n3422 = property on="trip1 8" class="Bool (strict)"("Boolean Text.Text"=w4423) -> ()  [unwired: 2 in, 2 out]
                }
                frame 126, Default {
                }
              }
            }
          }
          frame #1 {
            w4431 = TRUE ("Visible")
            n3423 = local read "S 91"() -> (w4448:string)
            n3424 = local read "S 90"() -> (w4447:string)
            n3425 = local read "S 88"() -> (w4446:string)
            n3426 = property on="File Path" class="Path"("Caption.Text"=w4447) -> ()  [unwired: 2 in, 2 out]
            n3427 = property on="SrvM CP" class="Bool (strict)"("Boolean Text.Text"=w4446) -> ()  [unwired: 2 in, 2 out]
            n3428 = local read "S 71"() -> (w4441:string)
            n3429 = local read "S 86"() -> (w4443:string)
            n3430 = local read "S 85"() -> (w4444:string)
            n3431 = local read "S 87"() -> (w4442:string)
            n3432 = local read "S 84"() -> (w4445:string)
            n3433 = local read "S 103"() -> (w4430:string)
            n3434 = local read "S 104"() -> (w4429:string)
            n3435 = property on="ENTER THE NEW PASSWORD" class="Str"("Caption.Text"=w4442) -> ()  [unwired: 2 in, 2 out]
            n3436 = property on="Password" class="Str"("Caption.Text"=w4444) -> ()  [unwired: 2 in, 2 out]
            n3437 = property on="ENTER CURRENT PASSWORD" class="Str"("Caption.Text"=w4443) -> ()  [unwired: 2 in, 2 out]
            n3438 = property on="EDIT" class="Bool (strict)"("Boolean Text.Text"=w4441) -> ()  [unwired: 2 in, 2 out]
            n3439 = property on="SAVE" class="Bool (strict)"("Boolean Text.Text"=w4445) -> ()  [unwired: 2 in, 2 out]
            n3440 = Build Array(w4430, w4429) -> (w4428:string[])
            n3441 = property on="Heater Button" class="Bool (strict)"("Strings [4]"=w4428) -> ()  [unwired: 2 in, 2 out]
            n3442 = property on="CH-HUMIDITY WET" class="DigNum (strict)"("Caption.Size to Text?"=w4431) -> ()  [unwired: 2 in, 2 out]
            n3443 = property on="CH-HUMIDITY DRY" class="DigNum (strict)"("Caption.Size to Text?"=w4431) -> ()  [unwired: 2 in, 2 out]
            n3444 = property on="CH-POWER -" class="DigNum (strict)"("Caption.Size to Text?"=w4431) -> ()  [unwired: 2 in, 2 out]
            n3445 = property on="CH-HEATER" class="DigNum (strict)"("Caption.Size to Text?"=w4431) -> ()  [unwired: 2 in, 2 out]
            n3446 = property on="CH-POWER +" class="DigNum (strict)"("Caption.Size to Text?"=w4431) -> ()  [unwired: 2 in, 2 out]
            n3447 = local read "S 92"() -> (w4440:string)
            n3448 = local read "S 93"() -> (w4439:string)
            n3449 = local read "S 105"() -> (w4426:string)
            n3450 = local read "S 106"() -> (w4425:string)
            n3451 = Build Array(w4440, w4439) -> ()  [unwired: 1 out]
            n3452 = Build Array(w4426, w4425) -> (w4427:string[])
            n3453 = local read "S 95"() -> (w4437:string)
            n3454 = local read "S 94"() -> (w4438:string)
            n3455 = local read "bs"() -> (w4453:string)
            n3456 = local read "as"() -> (w4454:string)
            n3457 = property on="Humidity" class="Bool (strict)"("Strings [4]"=w4427) -> ()  [unwired: 2 in, 2 out]
            n3458 = Concatenate Strings(w4453, "\r", w4454) -> ()  [unwired: 1 out]
            n3459 = property on="STROKE GAIN :" class="DigNum (strict)"("Caption.Text"=w4437) -> ()  [unwired: 2 in, 2 out]
            n3460 = property on="DISPLACEMENT :" class="DigNum (strict)"("Caption.Text"=w4438) -> ()  [unwired: 2 in, 2 out]
            n3461 = property on="Rh After" class="DigNum (strict)"("Caption.Size to Text?"=TRUE ("Caption.Size to Text")) -> ()  [unwired: 2 in, 2 out]
            n3462 = local read "S 48"() -> (w4477:string)
            n3463 = local read "S 50"() -> (w4475:string)
            n3464 = local read "S 51"() -> (w4474:string)
            n3465 = local read "S 49"() -> (w4476:string)
            n3466 = local read "S 52"() -> (w4473:string)
            n3467 = local read "as"() -> (w4458:string)
            n3468 = local read "bs"() -> (w4459:string)
            n3469 = local read "S 56"() -> (w4472:string)
            n3470 = local read "S 57"() -> (w4471:string)
            n3471 = local read "S 58"() -> (w4470:string)
            n3472 = local read "S 59"() -> (w4469:string)
            n3473 = property on="OPEN" class="Bool (strict)"("Boolean Text.Text"=w4473) -> ()  [unwired: 2 in, 2 out]
            n3474 = property on="OPEN 1" class="Bool (strict)"("Boolean Text.Text"=w4477) -> ()  [unwired: 2 in, 2 out]
            n3475 = property on="OPEN 2" class="Bool (strict)"("Boolean Text.Text"=w4476) -> ()  [unwired: 2 in, 2 out]
            n3476 = property on="OPEN 3" class="Bool (strict)"("Boolean Text.Text"=w4475) -> ()  [unwired: 2 in, 2 out]
            n3477 = property on="OPEN 4" class="Bool (strict)"("Boolean Text.Text"=w4474) -> ()  [unwired: 2 in, 2 out]
            n3478 = Concatenate Strings(w4459, "\r", w4458) -> ()  [unwired: 1 out]
            n3479 = local read "S 102"() -> (w4432:string)
            n3480 = property on="КОФ1" class="DigNum (strict)"("Caption.Text"=w4472) -> ()  [unwired: 2 in, 2 out]
            n3481 = local read "S 98"() -> (w4436:string)
            n3482 = local read "S 99"() -> (w4435:string)
            n3483 = local read "S 100"() -> (w4434:string)
            n3484 = local read "S 101"() -> (w4433:string)
            n3485 = property on="КОФ2" class="DigNum (strict)"("Caption.Text"=w4471) -> ()  [unwired: 2 in, 2 out]
            n3486 = property on="КОФ3" class="DigNum (strict)"("Caption.Text"=w4470) -> ()  [unwired: 2 in, 2 out]
            n3487 = property on="КОФ4" class="DigNum (strict)"("Caption.Text"=w4469) -> ()  [unwired: 2 in, 2 out]
            n3488 = local read "bs"() -> (w4457:string)
            n3489 = local read "as"() -> (w4456:string)
            n3490 = property on="CH-POWER +" class="DigNum (strict)"("Caption.Text"=w4436) -> ()  [unwired: 2 in, 2 out]
            n3491 = property on="CH-POWER -" class="DigNum (strict)"("Caption.Text"=w4435) -> ()  [unwired: 2 in, 2 out]
            n3492 = property on="CH-HEATER" class="DigNum (strict)"("Caption.Text"=w4434) -> ()  [unwired: 2 in, 2 out]
            n3493 = property on="CH-HUMIDITY DRY" class="DigNum (strict)"("Caption.Text"=w4433) -> ()  [unwired: 2 in, 2 out]
            n3494 = property on="CH-HUMIDITY WET" class="DigNum (strict)"("Caption.Text"=w4432) -> ()  [unwired: 2 in, 2 out]
            n3495 = local read "S 60"() -> (w4468:string)
            n3496 = local read "S 54"() -> (w4478:string)
            n3497 = Concatenate Strings(w4457, "\r", w4456) -> ()  [unwired: 1 out]
            n3498 = Concatenate Strings(w4478, w4468) -> ()  [unwired: 1 out]
            n3499 = local read "S 77"() -> (→"String 43":string)
            n3500 = local read "S 76"() -> (w4451:string)
            n3501 = local read "S 78"() -> (w4450:string)
            n3502 = local read "S 71"() -> (w4462:string)
            n3503 = local read "S 66"() -> (w4467:string)
            n3504 = local read "S 67"() -> (w4466:string)
            n3505 = local read "S 68"() -> (w4465:string)
            n3506 = local read "S 69"() -> (w4464:string)
            n3507 = local read "S 70"() -> (w4463:string)
            n3508 = property on="AIR TEMP" class="DigNum (strict)"("Caption.Text"=w4450) -> ()  [unwired: 2 in, 2 out]
            n3509 = property on="Set Strk" class="DigNum (strict)"("Caption.Text"=w4451) -> ()  [unwired: 2 in, 2 out]
            n3510 = property on="FRIC. FORCE :" class="DigNum (strict)"("Caption.Text"=w4467) -> ()  [unwired: 2 in, 2 out]
            n3511 = property on="TEMPERATURE :" class="DigNum (strict)"("Caption.Text"=w4466) -> ()  [unwired: 2 in, 2 out]
            n3512 = property on="SPEED OUT:" class="DigNum (strict)"("Caption.Text"=w4465) -> ()  [unwired: 2 in, 2 out]
            n3513 = property on="AIR TEMPERATURE :" class="DigNum (strict)"("Caption.Text"=w4464) -> ()  [unwired: 2 in, 2 out]
            n3514 = property on="HUMIDITY:" class="DigNum (strict)"("Caption.Text"=w4463) -> ()  [unwired: 2 in, 2 out]
            n3515 = property on="EDIT" class="Bool (strict)"("Boolean Text.Text"=w4462) -> ()  [unwired: 2 in, 2 out]
            n3516 = local read "S 79"() -> (w4449:string)
          }
          frame #2 {
          }
        }
        n3517 = local write "Lan flag"(10.0 ("Lan flag")) -> ()
      }
      frame Enabled {
      }
    }
    n3518 = Wait (ms)(milliseconds to wait=u32 2000) -> ()  [unwired: 1 out]
    n3519 = local read "Quit"() -> (w4252:bool)
  }
  n3520 = disable-structure shown="Disabled" {
    frame Disabled {
      n3521 = while {
        tunnel: [w4480] -> _
        i -> [w4480]
        stop <- w4479 continue-if-true
        n3522 = Wait (ms)(milliseconds to wait=u32 50) -> ()  [unwired: 1 out]
        n3523 = stacked-sequence {
          frame #0 {
            # "Controls Text color"
            # "Controls BG color"
            n3524 = property on="FILE" class="Str"("Text.Text Colors:Text Color"="SC  Text") -> ()  [unwired: 2 in, 2 out]
            n3525 = property on="Fuel Discription :" class="Str"("Text.Text Colors:Text Color"="SC  Text") -> ()  [unwired: 2 in, 2 out]
            n3526 = property on="tested by" class="Str"("Text.Text Colors:Text Color"="SC  Text") -> ()  [unwired: 2 in, 2 out]
            n3527 = property on="Remarks :" class="Str"("Text.Text Colors:Text Color"="SC  Text") -> ()  [unwired: 2 in, 2 out]
            n3528 = property class="DigNum (strict)"("Numeric Text.Text Colors:BG Color"="NC BG") -> ()  [unwired: 2 in, 2 out]
            n3529 = property class="DigNum (strict)"("Numeric Text.Text Colors:BG Color"="NC BG") -> ()  [unwired: 2 in, 2 out]
            n3530 = property class="DigNum (strict)"("Numeric Text.Text Colors:BG Color"="NC BG") -> ()  [unwired: 2 in, 2 out]
            n3531 = property class="DigNum (strict)"("Numeric Text.Text Colors:BG Color"="NC BG") -> ()  [unwired: 2 in, 2 out]
            n3532 = property class="DigNum (strict)"("Numeric Text.Text Colors:BG Color"="NC BG") -> ()  [unwired: 2 in, 2 out]
